vi "Matrix Invert Print Result.vi"() -> ()   [LabVIEW 2014, in "Arduino MatrixMath.lvlib"]
uses:
  <vilib>/Aledyne-TSXperts/Arduino Compatible Compiler for LabVIEW/addons/Arduino MatrixMath/Arduino MatrixMath.lvlib
  <vilib>/Aledyne-TSXperts/Arduino Compatible Compiler for LabVIEW/Arduino Compatible Compiler for LabVIEW.lvlib
panel:
  out "Success?":bool
  in  "A":sgl[](array[numeric])=[1.0, 0.0, 0.0, 1.0, 1.0, 0.0, 0.0, 0.0, 0.0]
  out "Error Out":errorcluster
  in  "Error In":errorcluster
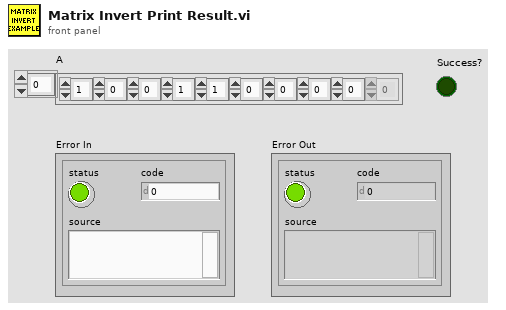
[diagram p1: front panel]
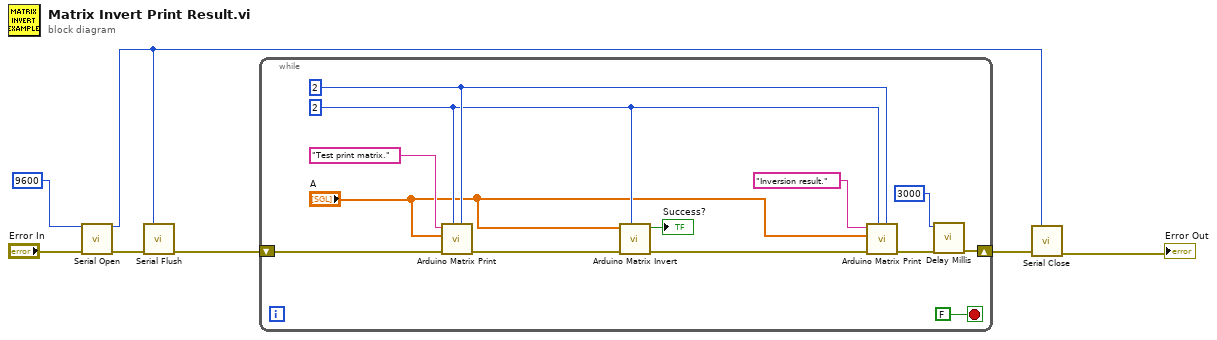
[diagram p0: block diagram]
diagram:
  n1 = call <vilib>:"Serial Open.vi"("Speed"=u32 9600, "error in (no error)"="Error In") -> ("Instance"=w1:u8, "error out"=w3:errorcluster)  [unwired: 12 in]
  n2 = call <vilib>:"Serial Flush.vi"("Instance"=w1, "error in (no error)"=w3) -> ("error out"=w2:errorcluster)  [unwired: 13 in]
  n3 = while {
    shift-right: [w16] -> w7
    shift-left: w2 -> [w19]
    stop <- FALSE stop-if-true
    w13 = u8 2 ("cols num.")
    w10 = u8 2 ("rows num.")
    n4 = call <vilib>:"Arduino Matrix Print.vi"("cols num."=w13, "rows num."=w10, "Error In"=w19, "A"="A", "Label"="Test print matrix.") -> ("Error Out"=w12:errorcluster)  [unwired: 6 in]
    n5 = call <vilib>:"Arduino Matrix Invert.vi"("rows num. A = (n x n)"=w10, "Error In"=w12, "A"="A") -> ("Error Out"=w11:errorcluster, "Success?"=→"Success?":bool)  [unwired: 7 in]
    n6 = call <vilib>:"Arduino Matrix Print.vi"("cols num."=w13, "rows num."=w10, "Error In"=w11, "A"="A", "Label"="Inversion result.") -> ("Error Out"=w15:errorcluster)  [unwired: 6 in]
    n7 = call <vilib>:"Delay Millis.vi"("error in (no error)"=w15, "delay"=u32 3000) -> ("error out"=w16:errorcluster)  [unwired: 9 in]
  }
  n8 = call <vilib>:"Serial Close.vi"("Instance"=w1, "error in (no error)"=w7) -> ("error out"=→"Error Out":errorcluster)  [unwired: 13 in]
